vi "Generate_position_one_dir.vi"(5 "HoppingDistance input":dbl, 7 "X Start input":dbl, 8 "Y P input":dbl, 9 "X P input":dbl, 10 "Scan Rate (um/s) input":dbl, 11 "X end input":dbl) -> (0 "Y velocity output":dbl, 2 "Y P output":dbl, 3 "X P output":dbl, 4 "X velocity output":dbl, 6 "Feedback type retraction output":u64)   [LabVIEW 2023]
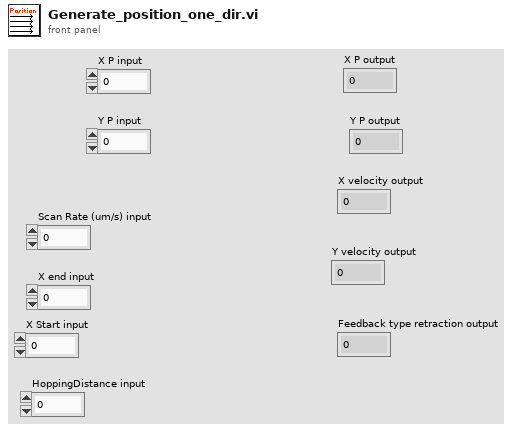
[diagram p1: front panel]
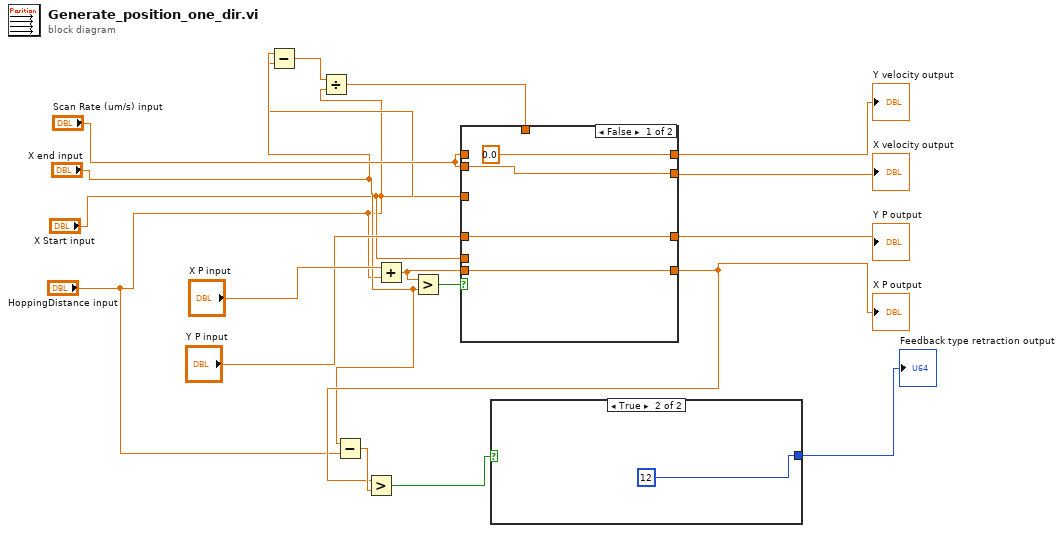
[diagram p0: block diagram]
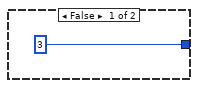
[diagram p2: hidden frame]
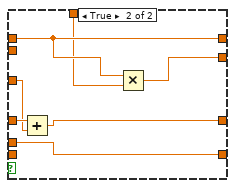
[diagram p3: hidden frame]
diagram:
  n1 = Subtract(x="X end input", y="X Start input") -> (x-y=w6:dbl)
  n2 = Divide(x=w6, y="HoppingDistance input") -> (x/y=w5:dbl)
  n3 = Subtract(x="X end input", y="HoppingDistance input") -> (x-y=w10:dbl)
  n4 = Add(x="X P input", y="HoppingDistance input") -> (x+y=w14:dbl)
  n5 = Greater?(x=w14, y="X end input") -> (0:w15:bool)
  n6 = case shown="False" w15 {
    tunnel: w14 -> [w19 _]
    tunnel: [w19 w25] -> w9
    tunnel: "Y P input" -> [w20 w28]
    tunnel: [w20 w27] -> w13
    tunnel: [w18 w23] -> w12
    tunnel: [0.0 w24] -> w11
    tunnel: "Scan Rate (um/s) input" -> [w18 _]
    tunnel: "HoppingDistance input" -> [_ w26]
    tunnel: "X Start input" -> [_ w25]
    tunnel: "Scan Rate (um/s) input" -> [_ w24]
    tunnel: w5 -> [_ w22]
    frame False {
    }
    frame True {
      n7 = Add(x=w28, y=w26) -> (x+y=w27:dbl)
      n8 = Multiply(x=w24, y=w22) -> (x*y=w23:dbl)
    }
  }
  "X P output" <- w9
  "Y P output" <- w13
  "X velocity output" <- w12
  "Y velocity output" <- w11
  n9 = Greater?(x=w9, y=w10) -> (0:w7:bool)
  n10 = case shown="True" w7 {
    tunnel: [u64 3 u64 12] -> w8
    frame False {
    }
    frame True {
    }
  }
  "Feedback type retraction output" <- w8
